vi "_CSTK_Button_Icon_EventUpdateControlView.vi"(6 "调用方":string, 7 "UpdateDrawArea":bool, 8 "错误输入（无错误）":errorcluster, 9 "DrawAreaSize":T1, 10 "BGImage":picture, 11 "用户事件输入":refnum<user-event>) -> (0 "错误输出":errorcluster, 3 "用户事件输出":refnum<user-event>)   [LabVIEW 2015, in "CSTK_Button_Icon.xctl"]
uses:
  CSTK_Button_Icon.xctl
  TypeDefinitions/_CSTK_Button_Icon_EventData.ctl
  <vilib>/Utility/miscctls.llb/LVBoundsTypeDef.ctl
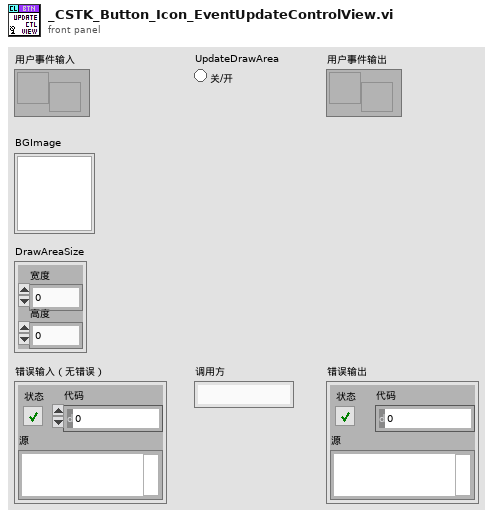
[diagram p1: front panel]
types:
  T1 = typedef "LVBoundsTypeDef.ctl" = cluster{"Width":u32, "Height":u32}
  T2 = typedef "CSTK_Button_Icon.xctl/_CSTK_Button_Icon_EventData.ctl" = cluster{"BGImage":picture, "DrawAreaSize":T1, "UpdateDrawArea":bool, "调用方":string}
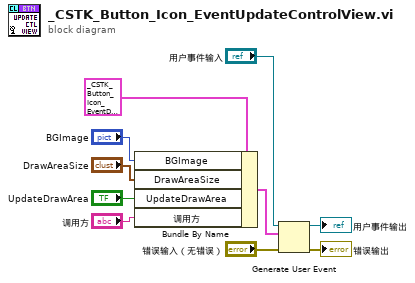
[diagram p0: block diagram]
diagram:
  n1 = Bundle By Name(cluster=T2 {"BGImage"=bytes[0], "DrawAreaSize"={"Width"=0, "Height"=0}, "UpdateDrawArea"=FALSE, "调用方"=""} ("事件数据"), "BGImage"="BGImage", "DrawAreaSize"="DrawAreaSize", "UpdateDrawArea"="UpdateDrawArea", "调用方"="调用方") -> (w10:T2)
  n2 = Generate User Event(user event="用户事件输入", event data cluster=w10, error in="错误输入（无错误）") -> (user event out=→"用户事件输出":refnum<user-event>, error out=→"错误输出":errorcluster)  [unwired: 1 in]
